vi "1.4.2-Encoder Integration.vi"(0 "Encoder B":bool, 5 "Encoder A":bool, 9 "Encoder A Old":bool, 11 "Encoder B Old":bool, 13 "Encoder Index":bool) -> (3 "Count Delta":i32, 4 "The Encoder Changed":bool, 6 "Count Zeroed at Index":i32, 8 "Encoder A Old (sReg)":bool, 10 "Encoder B Old (sReg)":bool, 14 "Current count":i32)   [LabVIEW 2010]
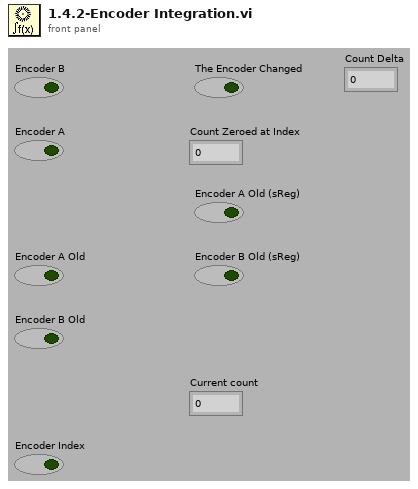
[diagram p1: front panel]
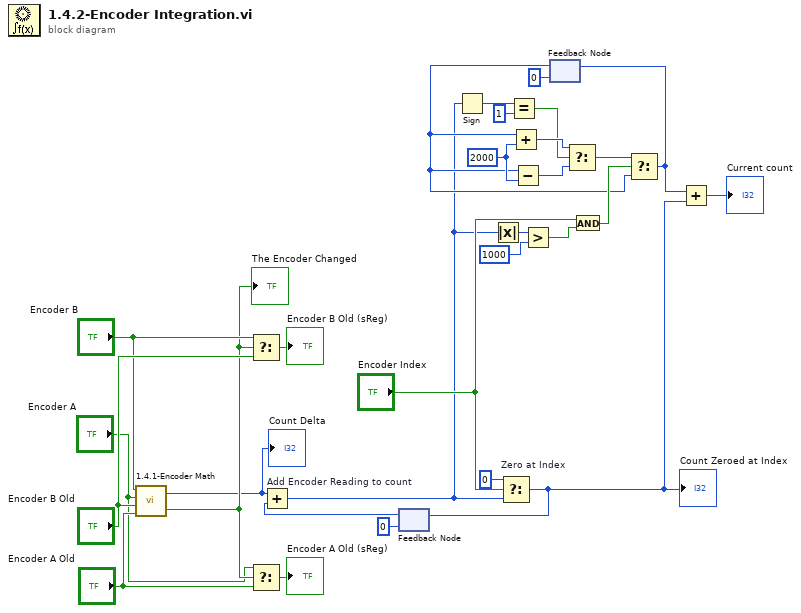
[diagram p0: block diagram]
diagram:
  w21 = 2000 ("y")
  n1 = call "1.4.1-Encoder Math.vi"("Encoder A_old"="Encoder A Old", "Encoder B_old"="Encoder B Old", "Encoder A_new"="Encoder A", "Encoder B_new"="Encoder B") -> ("The Encoder Changed"=w26:bool, "Change in Encoder Value"=w1:i32)
  "The Encoder Changed" <- w26
  "Count Delta" <- w1
  n2 = Select(t="Encoder B", s=w26, f="Encoder B Old") -> (s? t:f=→"Encoder B Old (sReg)":bool)
  n3 = Select(t="Encoder A", s=w26, f="Encoder A Old") -> (s? t:f=→"Encoder A Old (sReg)":bool)
  n4 = feedback #1(0) -> (w9:i32)
  n5 = Add "Add Encoder Reading to count"(x=w1, y=w9) -> (x+y=w2:i32)
  n6 = Sign(1:w2) -> (0:w18:i32)
  n7 = Absolute Value(x=w2) -> (abs(x)=w14:i32)
  n8 = Select "Zero at Index"(t=0 ("Zero at Index"), s="Encoder Index", f=w2) -> (s? t:f=w4:i32)
  "Count Zeroed at Index" <- w4
  n9 = feedback-in #1(w4) -> ()
  n10 = Equal?(x=w18, y=1) -> (x = y?=w17:bool)
  n11 = Greater?(x=w14, y=1000) -> (0:w12:bool)
  n12 = feedback #2(0) -> (w7:i32)
  n13 = Add(x=w7, y=w21) -> (x+y=w20:i32)
  n14 = Subtract(x=w7, y=w21) -> (x-y=w19:i32)
  n15 = Select(t=w20, s=w17, f=w19) -> (s? t:f=w15:i32)
  n16 = And(x="Encoder Index", y=w12) -> (x .and. y?=w10:bool)
  n17 = Select(t=w15, s=w10, f=w7) -> (s? t:f=w5:i32)
  n18 = feedback-in #2(w5) -> ()
  n19 = Add(x=w5, y=w4) -> (x+y=→"Current count":i32)
